vi "RS232C_WaitReady_re.vi"(2 "Delimiter":string="\\r\\n", 3 "PortNumber":i32) -> (0 "OK Done":bool, 1 "String Received":string)   [LabVIEW 2016]
panel:
  # "Port Number 0=COM1"
  # "Send '!:'+delimiter and wait for 'R'+delimiter.\nAn Error occurs when timed out."
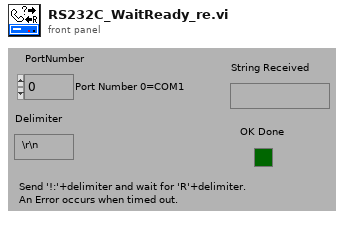
[diagram p1: front panel]
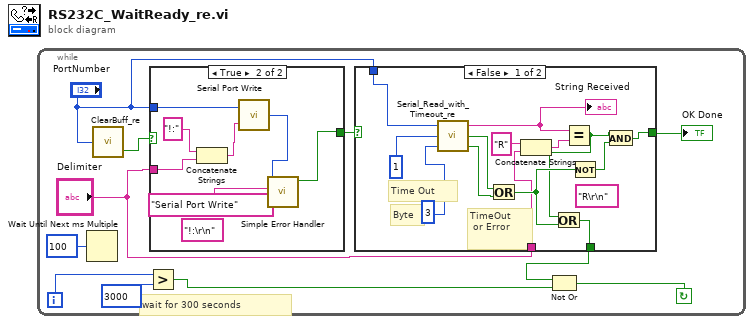
[diagram p0: block diagram]
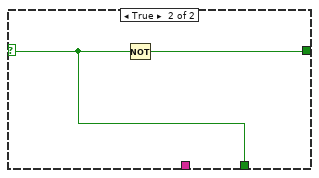
[diagram p2: hidden frame]
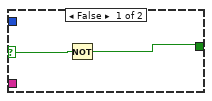
[diagram p3: hidden frame]
diagram:
  n1 = while {
    i -> [w8]
    stop <- w5 continue-if-true
    # "wait for 300 seconds"
    n2 = Wait Until Next ms Multiple(millisecond multiple=100) -> ()  [unwired: 1 out]
    n3 = call "ClearBuff_re.vi"("PortNumber"="PortNumber") -> ("OK Done"=w2:bool)  [unwired: 1 out]
    n4 = Greater?(x=w8, y=3000) -> (0:w6:bool)
    n5 = case shown="True" w2 {
      selector: w2 -> [w29 _]
      tunnel: "PortNumber" -> [_ w36]
      tunnel: [w28 w33] -> w11
      tunnel: "Delimiter" -> [_ w31]
      frame False {
        n6 = Not(x=w29) -> (.not. x?=w28:bool)
      }
      frame True {
        (unwired) "!:\r\n"
        n7 = Concatenate Strings("!:", w31) -> (w30:string)
        n8 = call <vilib>:"Serial Port Write.vi"("string to write"=w30, "port number"=w36) -> ("error code"=w34:i32)
        n9 = call <vilib>:"Simple Error Handler.vi"("error code (no error:0)"=w34, "error source (\" \")"="Serial Port Write") -> ("error?"=w33:bool)  [unwired: 2 in, 5 out]
      }
    }
    n10 = case shown="False" w11 {
      selector: w11 -> [_ w26]
      tunnel: "PortNumber" -> [w23 _]
      tunnel: [w20 w26] -> w7
      tunnel: [w16 w27] -> w4
      tunnel: "Delimiter" -> [w12 _]
      frame False {
        (unwired) "R\r\n"
        # "TimeOut\n or Error"
        # "Byte"
        # "Time Out"
        n11 = call "Serial_Read_with_Timeout_re.vi"("Bytes to Read"=3, "Timeout Limit"=1, "Port Number"=w23) -> ("Error Out"=w21:bool, "Timeout"=w22:bool, "Serial Read"=w19:string)
        "String Received" <- w19
        n12 = Or(x=w22, y=w21) -> (x .or. y?=w17:bool)
        n13 = Concatenate Strings("R", w12) -> (w14:string)
        n14 = Equal?(x=w19, y=w14) -> (x = y?=w15:bool)
        n15 = Or(x=w15, y=w17) -> (x .or. y?=w20:bool)
        n16 = Not(x=w17) -> (.not. x?=w18:bool)
        n17 = And(x=w15, y=w18) -> (x .and. y?=w16:bool)
      }
      frame True {
        n18 = Not(x=w26) -> (.not. x?=w27:bool)
      }
    }
    "OK Done" <- w4
    n19 = Not Or(1:w6, 2:w7) -> (0:w5:bool)
  }
